vi "Stop Module.vi"(8 "error in (no error)":errorcluster, 11 "Origin":string) -> (0 "error out":errorcluster)   [LabVIEW 2014, in "Chart Module.lvlib"]
uses:
  Chart Module.lvlib
  Stop Argument--cluster.ctl
  <vilib>/event_ctls.llb/usereventprio.ctl
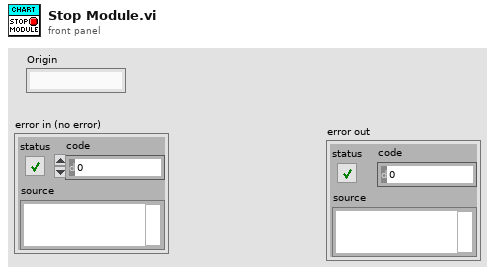
[diagram p1: front panel]
types:
  T1 = typedef "usereventprio.ctl" = enum32{"high priority", "normal priority"}
  T2 = typedef "Chart Module.lvlib/Stop Argument--cluster.ctl" = cluster{"Origin":string, "Exit via Stop Module Req?":bool}
  T3 = typedef "Chart Module.lvlib/Request Events--cluster.ctl" = cluster{"Stop Module":refnum<user-event>, "Show Panel":refnum<user-event>, "Hide Panel":refnum<user-event>}
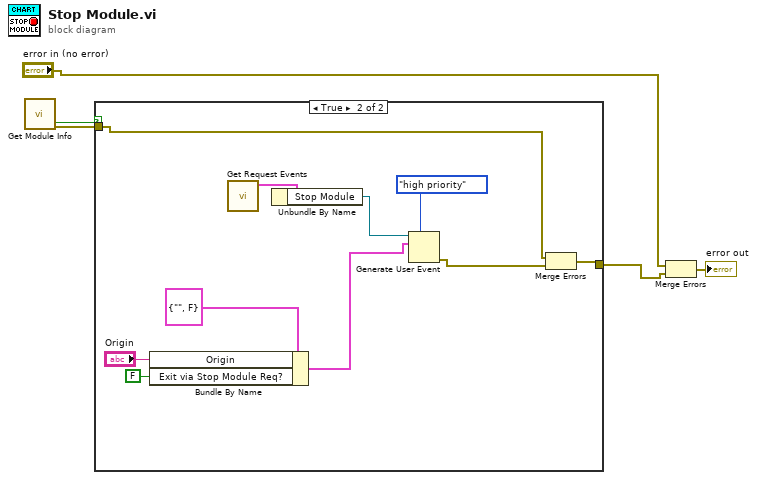
[diagram p0: block diagram]
diagram:
  n1 = call "Get Module Info.vi"() -> ("error out"=w2:errorcluster, "isModuleRunning?"=w5:bool)  [unwired: 8 in, 2 out]
  n2 = case shown="True" w5 {
    tunnel: [w6 w9] -> w3
    tunnel: w2 -> [w6 w8]
    frame False {
    }
    frame True {
      n3 = Bundle By Name(cluster=T2 {"Origin"="", "Exit via Stop Module Req?"=FALSE} ("Stop Argument"), "Origin"="Origin", "Exit via Stop Module Req?"=FALSE) -> (w11:T2)
      n4 = call "Get Request Events.vi"() -> ("Request Events"=w16:T3)  [unwired: 10 in, 1 out]
      n5 = Unbundle By Name(w16) -> ("Stop Module"=w15:refnum<user-event>)
      n6 = Generate User Event(priority (normal)=usereventprio."high priority", user event=w15, event data cluster=w11) -> (error out=w7:errorcluster)  [unwired: 1 in, 1 out]
      n7 = Merge Errors(w8, w7) -> (w9:errorcluster)
    }
  }
  n8 = Merge Errors("error in (no error)", w3) -> (→"error out":errorcluster)
